vi "PixData Duplicate 10x.vi"(8 "Width":i16, 9 "Height":i16, 11 "PixData In":u8[](array[numeric])) -> (0 "Output Width":i16, 1 "Output Height":i16, 3 "PixData Out":u8[](array[numeric]))   [LabVIEW 2013]
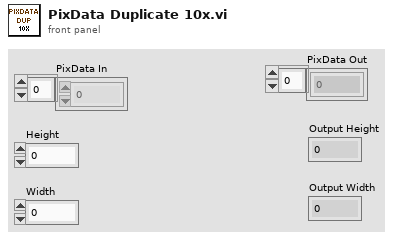
[diagram p1: front panel]
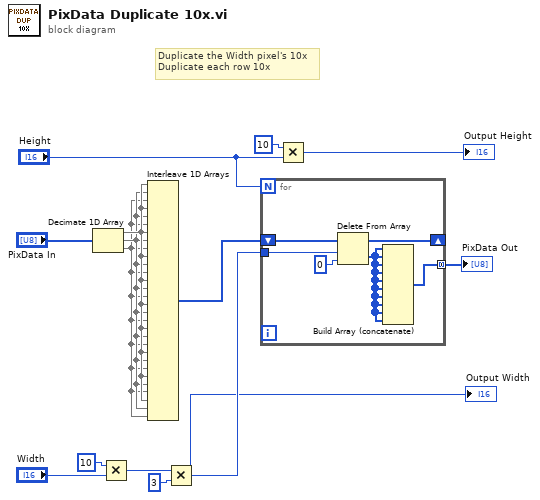
[diagram p0: block diagram]
diagram:
  # "Duplicate the Width pixel's 10x\nDuplicate each row 10x"
  n1 = Decimate 1D Array("PixData In") -> (w3:u8[], w2:u8[], w1:u8[])
  n2 = Multiply(x=i16 10, y="Width") -> (x*y=w12:i16)
  "Output Width" <- w12
  n3 = Interleave 1D Arrays(w3, w2, w1, w3, w2, w1, w3, w2, w1, w3, w2, w1, w3, w2, w1, w3, w2, w1, w3, w2, w1, w3, w2, w1, w3, w2, w1, w3, w2, w1) -> (w7:u8[])
  n4 = Multiply(x=w12, y=i16 3) -> (x*y=w14:i16)
  n5 = for {
    N: "Height" -> [_]
    tunnel: w14 -> [w19]
    shift-right: [w18] -> _
    shift-left: w7 -> [w17]
    tunnel: [w16] -> w8 mode=concatenating
    n6 = Delete From Array(array=w17, length=w19, index=0) -> (deleted portion=w15:u8[], array with subset deleted=w18:u8[])
    n7 = Build Array (concatenate)(w15, w15, w15, w15, w15, w15, w15, w15, w15, w15) -> (w16:u8[])
  }
  "PixData Out" <- w8
  n8 = Multiply(x=i16 10, y="Height") -> (x*y=→"Output Height":i16)
